vi "ExperimentSettingsMenu.vi"(0 "Enable":bool=TRUE, 1 "Default Group ID":u16(ring) items=["CCLDAS"=1, "LASP"=2, "CU"=3, "NLSI"=4, "LDEX"=5, "Heidelberg"=6], 2 "sub vi?":bool, 5 "error in (no error)":errorcluster, 6 "Default Experiment Name":string caption="Please Enter Tags:", 8 "default Experiment Description":string caption="Please Enter Experiment Description:") -> (13 "Update":bool caption="OK2", 14 "Cancel 2":bool caption="Cancel", 15 "Please Enter Experiment Description:":string, 16 "Please Enter Tags:":string, 17 "Please Enter Group ID":dbl format="%#g", 18 "New":bool caption="OK", 19 "error out":errorcluster)   [LabVIEW 2013]
doc: "Displays a standard dialog box that prompts users to enter information, such as a user name and password.\n--------------------\n\nThis Express VI is configured as follows:\n\nMessage to Display to the User:Please Enter Experiment Settings Information For Database Storage.\nThe inputs are: \nNumber: Please Enter Group ID\nText Entry Box: Please Enter Tags:\nText Entry Box: Please Enter Experiment Description:"
uses:
  <vilib>/Utility/miscctls.llb/LVPointTypeDef.ctl
  <vilib>/addons/database/Connection.llb/Conn Execute.vi
  <vilib>/addons/database/Recordset.llb/Rec Fetch Recordset Data (R).vi
  <vilib>/addons/database/Recordset.llb/Rec Destroy - Connection.vi
  <vilib>/addons/database/_DB Variant To Data/Database Variant To Data.xnode
  <vilib>/addons/database/NI_Database_API.lvlib
panel:
  in  "Add New Group":bool caption="OK2"
  out "Default Experiment Name 2":string caption="Please Enter Tags:"
  out "default Experiment Description 2":string caption="Please Enter Experiment Description:"
  out "Default Group ID 2":u16(ring) items=["CCLDAS"=1, "LASP"=2, "CU"=3, "NLSI"=4, "LDEX"=5, "Heidelberg"=6]
  in  "Please Select Experiment Group:":u16(ring) items=["Ablation Exp 4"=30, "Ablation Exp 3"=29, "Ejecta"=28, "Stanford"=27, "Ice Target"=26, "PVDF"=25, "Ablation Exp 2"=24, "Ablation Exp"=23, "Zoltan Dust Detectors"=22, "Small Acc Dust Type Testing"=21, "Todd Bradley Florida Group"=20, "HyperSuda"=19, "New Group Name"=18, "ODINSun"=17, "Ejecta Experiments 2014"=16, "Mehoke Foils"=15, "LDEX"=14, "Solar Cell"=13, "Eric Christian"=12, "STEREO"=11, "Neutral Gas"=10, "Maintenance"=9, "Evans little thingy"=8, "Keith the Drake"=7, "David Malaspina"=6, "November Lightflash"=5, "Throop Foils"=4, "NDA"=3, "Anna Spectrometer"=2, "June Lightflash"=1]
  in  "Please Enter an Experiment Description:":string caption="Please Enter Experiment Description:"
  in  "OK2":bool
  in  "Cancel":bool
  in  "Please Enter an Experiment Name:":string caption="Please Enter Tags:"
  in  "OK1":bool
  # "Please Enter Experiment Settings Information For Storage in the CCLDAS Database."
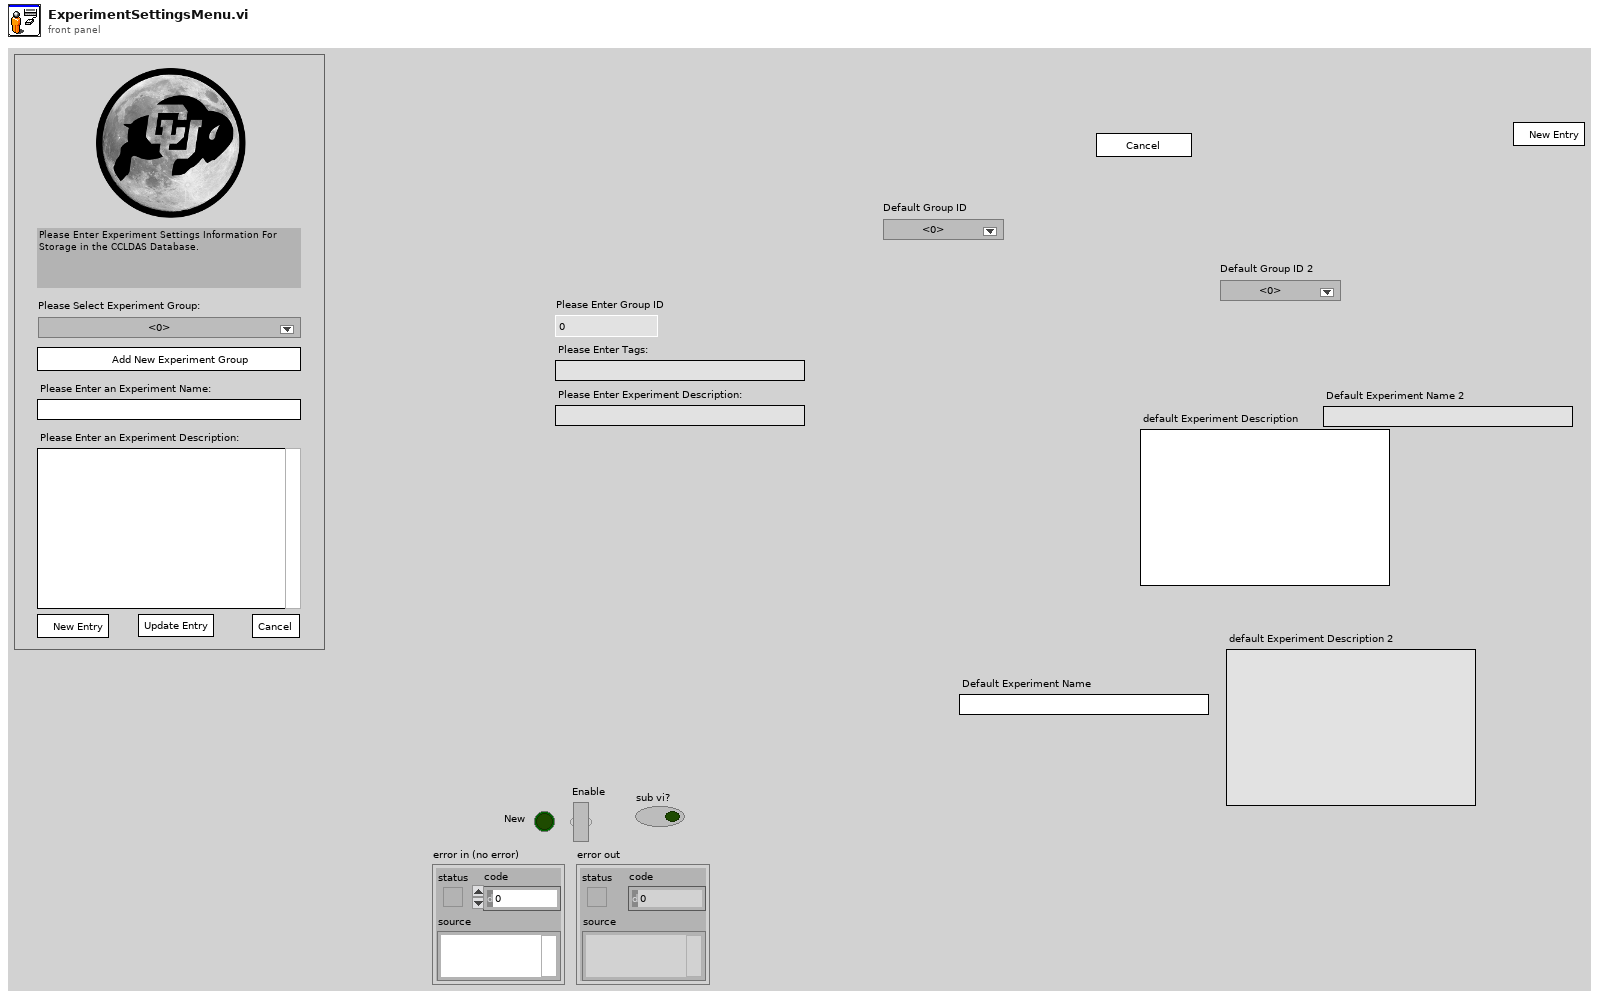
[diagram p1: front panel]
types:
  T1 = typedef "LVPointTypeDef.ctl" = cluster{"Horizontal":i16, "Vertical":i16}
  T2 = enum32{"Invalid", "Standard", "Closed", "Hidden", "Minimized", "Maximized"}
  T3 = typedef "NI_Database_API.lvlib/Conn ObjectReference.ctl" = refnum<k1>
  T4 = typedef "NI_Database_API.lvlib/Rec ObjectReference.ctl" = refnum<k1>
  T5 = cluster{"Input Name":string, "Input Data Type":i32}
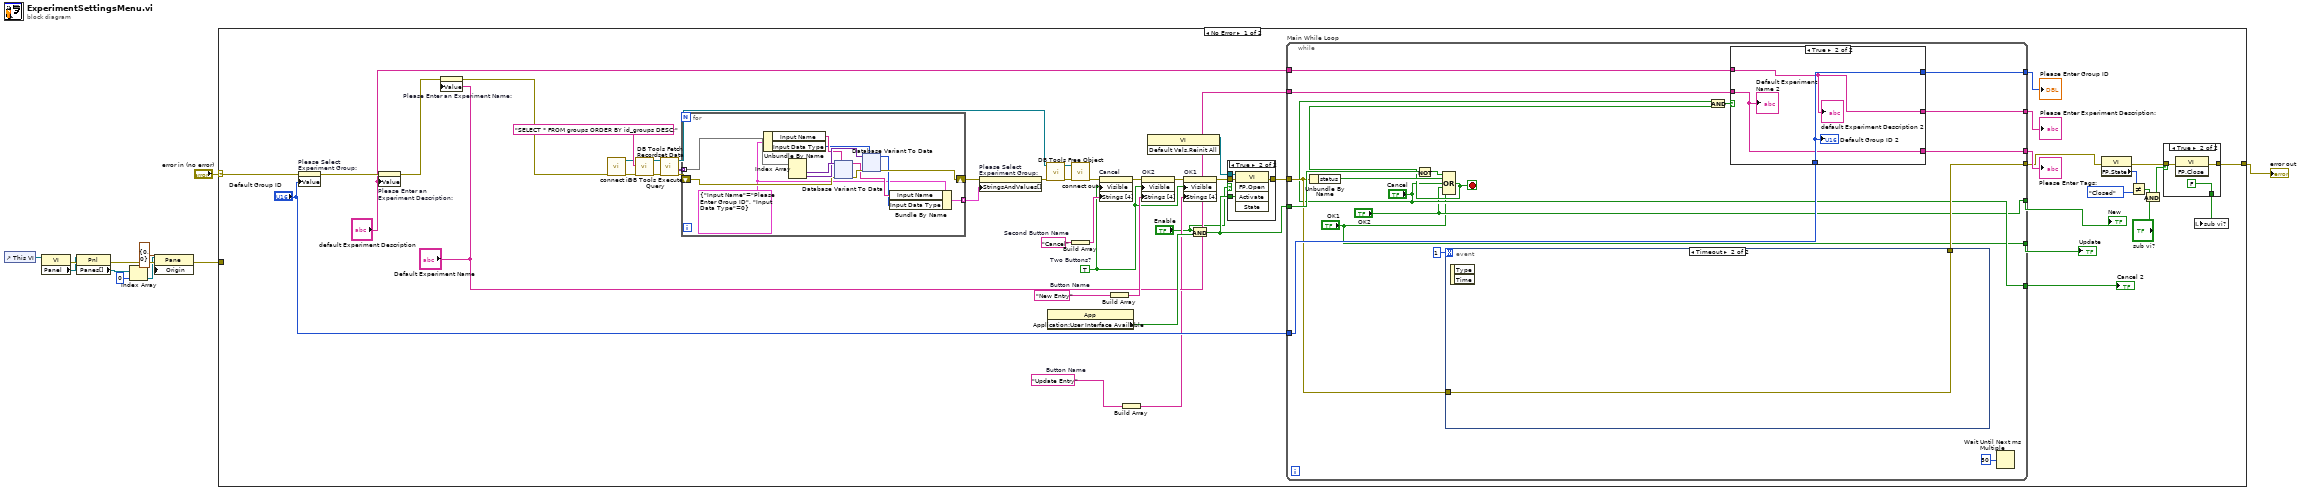
[diagram p0: block diagram]
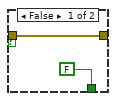
[diagram p2: hidden frame]
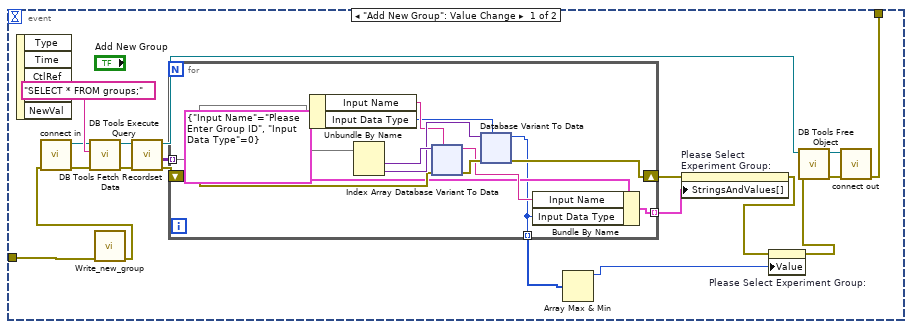
[diagram p4: hidden frame]
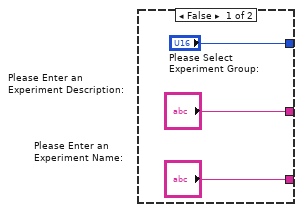
[diagram p5: hidden frame]
diagram:
  n1 = control-ref of="This VI"() -> (w9:refnum<vi>)
  n2 = property class="VI"(reference=w9) -> (error out=w8:errorcluster, "Panel"=w7:refnum<vi>)  [unwired: 1 in, 1 out]
  n3 = property class="Pnl"(reference=w7, error in=w8) -> (error out=w6:errorcluster, "Panes[]"=w5:refnum<vi>[])  [unwired: 1 out]
  n4 = Index Array(array=w5, index=0) -> (element=w3:refnum<vi>)
  n5 = property class="Pane"(reference=w3, error in=w6, "Origin"=T1 {"Horizontal"=0, "Vertical"=0}) -> (error out=w1:errorcluster)  [unwired: 1 out]
  n6 = case shown="No Error" "error in (no error)" {
    selector: "error in (no error)" -> [w37 w269]
    tunnel: [w25 w269] -> w10
    tunnel: w1 -> [_ _]
    frame No Error {
      w28 = "Update Entry"  # Button Name
      w42 = "Cancel"  # Second Button Name
      w44 = "New Entry"  # Button Name
      w29 = TRUE  # Two Buttons?
      n7 = property on="Please Select Experiment Group:" class="Ring (strict)"(error in=w37, "Value"="Default Group ID") -> (error out=w36:errorcluster)  [unwired: 1 in, 1 out]
      n8 = property on="Please Enter an Experiment Description:" class="Str"(error in=w36, "Value"="default Experiment Description") -> (error out=w35:errorcluster)  [unwired: 1 in, 1 out]
      n9 = property on="Please Enter an Experiment Name:" class="Str"(error in=w35, "Value"="Default Experiment Name") -> (error out=w34:errorcluster)  [unwired: 1 in, 1 out]
      n10 = call "connect in.vi"("error in (no error)"=w34) -> ("error out"=w50:errorcluster, "Database Connection"=w49:T3)  [unwired: 6 in, 1 out]
      n11 = call-poly <vilib>:"DB Tools Execute Query.vi"("error in (no error)"=w50, "SQL query"="SELECT * FROM groups ORDER BY id_groups DESC;", "connection reference"=w49) -> ("error out"=w52:errorcluster, "recordset reference"=w51:T4)  [unwired: 5 in]
      n12 = call-poly <vilib>:"DB Tools Fetch Recordset Data.vi"("error in (no error)"=w52, "recordset reference"=w51) -> ("error out"=w59:errorcluster, "recordset data"=w58:variant[][], "recordset reference out"=w53:T4)  [unwired: 3 in]
      n13 = for {
        tunnel: w58 -> [w84] mode=indexing
        shift-right: [w79] -> w60
        shift-left: w59 -> [w80]
        tunnel: [w78] -> w62 mode=indexing
        w73 = T5 {"Input Name"="Please Enter Group ID", "Input Data Type"=0}
        n14 = Unbundle By Name(w73) -> ("Input Name"=w77:string, "Input Data Type"=w74:i32)
        n15 = Index Array(array=w84) -> (element #1=w83:variant, element #2=w82:variant)  [unwired: 2 in]
        n16 = xnode "Database Variant To Data"("database variant"=w83, "error in"=w80, "type"=w77) -> ("data"=w76:string, "error out"=w81:errorcluster)
        n17 = xnode "Database Variant To Data"("database variant"=w82, "error in"=w81, "type"=w74) -> ("data"=w75:i32, "error out"=w79:errorcluster)
        n18 = Bundle By Name(cluster=w73, "Input Name"=w76, "Input Data Type"=w75) -> (w78:T5)
      }
      n19 = property on="Please Select Experiment Group:" class="Ring (strict)"(error in=w60, "StringsAndValues[]"=w62) -> (error out=w61:errorcluster)  [unwired: 1 in, 1 out]
      n20 = call-poly <vilib>:"DB Tools Free Object.vi"("error in (no error)"=w61, "recordset reference"=w53) -> ("error out"=w54:errorcluster, "connection reference"=w55:T3)  [unwired: 8 in]
      n21 = property class="App"() -> ("Application:User Interface Available"=w45:bool)  [unwired: 2 in, 2 out]
      n22 = call "connect out.vi"("error in (no error)"=w54, "connection reference"=w55) -> ("error out"=w56:errorcluster)  [unwired: 9 in]
      n23 = Build Array(w42) -> (w41:string[])
      n24 = property on="Cancel" class="Bool"(error in=w56, "Visible"=w29, "Strings [4]"=w41) -> (error out=w39:errorcluster)  [unwired: 1 in, 1 out]
      n25 = Build Array(w44) -> (w43:string[])
      n26 = Build Array(w28) -> (w27:string[])
      n27 = property on="OK2" class="Bool"(error in=w39, "Visible"=w29, "Strings [4]"=w43) -> (error out=w40:errorcluster)  [unwired: 1 in, 1 out]
      n28 = invoke class="VI" method="Default Vals.Reinit All"() -> (reference out=w21:refnum<vi>)  [unwired: 3 in, 2 out]
      n29 = property on="OK1" class="Bool"(error in=w40, "Visible"=w29, "Strings [4]"=w27) -> (error out=w24:errorcluster)  [unwired: 1 in, 1 out]
      n30 = And(x="Enable", y=w45) -> (x .and. y?=w22:bool)
      n31 = case shown="True" "Enable" {
        tunnel: w24 -> [w68 w72]
        tunnel: [w68 w71] -> w23
        tunnel: w22 -> [_ w70]
        tunnel: w21 -> [_ w69]
        frame False {
        }
        frame True {
          n32 = invoke class="VI" method="FP.Open"(reference=w69, error in=w72, "Activate"=w70) -> (error out=w71:errorcluster)  [unwired: 2 in, 4 out]
        }
      }
      n33 = while "Main While Loop" {
        tunnel: ["OK2"] -> w38
        tunnel: w22 -> [w165]
        tunnel: w23 -> [w154]
        tunnel: [w153] -> w19
        tunnel: [w160] -> w46
        tunnel: [w162] -> w47
        tunnel: [w161] -> w48
        tunnel: "Default Experiment Name" -> [w157]
        tunnel: "default Experiment Description" -> [w156]
        tunnel: "Default Group ID" -> [w155]
        tunnel: ["Cancel"] -> w30
        tunnel: ["OK1"] -> w26
        stop <- w158 stop-if-true
        n34 = Unbundle By Name(w154) -> ("status"=w163:bool)
        n35 = Not(x=w165) -> (.not. x?=w164:bool)
        n36 = Compound Arithmetic op=OR(w164, w163, "Cancel", "OK2", "OK1") -> (w158:bool)
        n37 = event shown="[1] Timeout" {
          selector: _ -> [_ _]
          dyn-events: _ -> [_ _]
          timeout: 1 -> [_ _]
          tunnel: w154 -> [w172 w262]
          tunnel: [w171 w262] -> w153
          event "Add New Group": Value Change {
            n38 = event-data() -> ()  [unwired: 1 in, 5 out]
            n39 = call "Write_new_group.vi"("error in (no error)"=w172) -> ("error out"=w173:errorcluster)  [unwired: 9 in, 1 out]
            n40 = call "connect in.vi"("error in (no error)"=w173) -> ("error out"=w175:errorcluster, "Database Connection"=w174:T3)  [unwired: 6 in, 1 out]
            n41 = call-poly <vilib>:"DB Tools Execute Query.vi"("error in (no error)"=w175, "SQL query"="SELECT * FROM groups;", "connection reference"=w174) -> ("error out"=w177:errorcluster, "recordset reference"=w176:T4)  [unwired: 5 in]
            n42 = call-poly <vilib>:"DB Tools Fetch Recordset Data.vi"("error in (no error)"=w177, "recordset reference"=w176) -> ("error out"=w183:errorcluster, "recordset data"=w182:variant[][], "recordset reference out"=w178:T4)  [unwired: 3 in]
            n43 = for {
              tunnel: w182 -> [w197] mode=indexing
              shift-right: [w192] -> w184
              shift-left: w183 -> [w193]
              tunnel: [w191] -> w185 mode=indexing
              tunnel: [w186] -> w168 mode=indexing
              w187 = T5 {"Input Name"="Please Enter Group ID", "Input Data Type"=0}
              n44 = Unbundle By Name(w187) -> ("Input Name"=w190:string, "Input Data Type"=w188:i32)
              n45 = Index Array(array=w197) -> (element #1=w196:variant, element #2=w195:variant)  [unwired: 2 in]
              n46 = xnode "Database Variant To Data"("database variant"=w196, "error in"=w193, "type"=w190) -> ("data"=w189:string, "error out"=w194:errorcluster)
              n47 = xnode "Database Variant To Data"("database variant"=w195, "error in"=w194, "type"=w188) -> ("data"=w186:i32, "error out"=w192:errorcluster)
              n48 = Bundle By Name(cluster=w187, "Input Name"=w189, "Input Data Type"=w186) -> (w191:T5)
            }
            n49 = Array Max & Min(array=w168) -> (max value=w167:i32)  [unwired: 3 out]
            n50 = property on="Please Select Experiment Group:" class="Ring (strict)"(error in=w184, "StringsAndValues[]"=w185) -> (error out=w170:errorcluster)  [unwired: 1 in, 1 out]
            n51 = property on="Please Select Experiment Group:" class="Ring (strict)"(error in=w170, "Value"=w167) -> (error out=w169:errorcluster)  [unwired: 1 in, 1 out]
            n52 = call-poly <vilib>:"DB Tools Free Object.vi"("error in (no error)"=w169, "recordset reference"=w178) -> ("error out"=w179:errorcluster, "connection reference"=w180:T3)  [unwired: 8 in]
            n53 = call "connect out.vi"("error in (no error)"=w179, "connection reference"=w180) -> ("error out"=w171:errorcluster)  [unwired: 9 in]
          }
          event Timeout {
            n54 = event-data() -> ()  [unwired: 1 in, 2 out]
          }
        }
        n55 = And(x="Cancel", y=w158) -> (x .and. y?=w159:bool)
        n56 = case shown="True" w159 {
          tunnel: ["Please Enter an Experiment Name:" w266] -> w162
          tunnel: ["Please Enter an Experiment Description:" w267] -> w161
          tunnel: ["Please Select Experiment Group:" w268] -> w160
          tunnel: w157 -> [_ w266]
          tunnel: w156 -> [_ w267]
          tunnel: w155 -> [_ w268]
          frame False {
          }
          frame True {
            "Default Group ID 2" <- w268
            "default Experiment Description 2" <- w267
            "Default Experiment Name 2" <- w266
          }
        }
        n57 = Wait Until Next ms Multiple(millisecond multiple=u32 50) -> ()  [unwired: 1 out]
      }
      "New" <- w38
      "Please Enter Group ID" <- w46
      "Please Enter Tags:" <- w47
      "Please Enter Experiment Description:" <- w48
      "Cancel 2" <- w30
      "Update" <- w26
      n58 = property class="VI"(error in=w19) -> (error out=w18:errorcluster, "FP.State"=w17:T2)  [unwired: 1 in, 1 out]
      n59 = Not Equal?(x=w17, y=T2."Closed") -> (x != y?=w13:bool)
      n60 = And(x=w13, y="sub vi?") -> (x .and. y?=w14:bool)
      n61 = case shown="True" w14 {
        tunnel: [w64 w67] -> w25
        tunnel: w18 -> [w64 w66]
        tunnel: [FALSE ("sub vi?") FALSE ("sub vi?")] -> w12
        frame False {
        }
        frame True {
          n62 = invoke class="VI" method="FP.Close"(error in=w66) -> (error out=w67:errorcluster)  [unwired: 2 in, 2 out]
        }
      }
      n63 = local write "sub vi?"(w12) -> ()
    }
    frame Error {
    }
  }
  "error out" <- w10
